vi "SetPropellerOutputPin.vi"(6 "error in (no error)":errorcluster, 8 "Pin Number":dbl, 9 "Value":bool, 10 "Dir":bool, 11 "SerialPortRef":T1) -> (0 "error out":errorcluster, 3 "SerialPortRef 2":T1)   [LabVIEW 2015]
uses:
  <vilib>/Rock Robotics/WPI/SerialPort/WPI_SerialPortRef.ctl
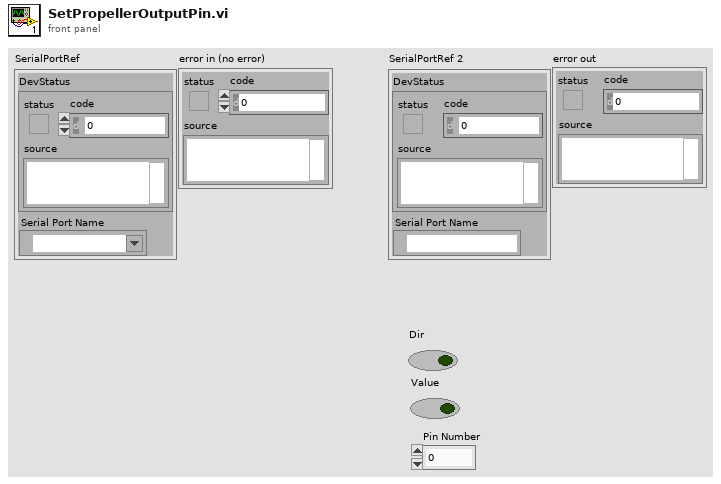
[diagram p1: front panel]
types:
  T1 = typedef "WPI_SerialPortRef.ctl" = cluster{"DevStatus":errorcluster, "Serial Port Name":refnum<visa-resource-name>}
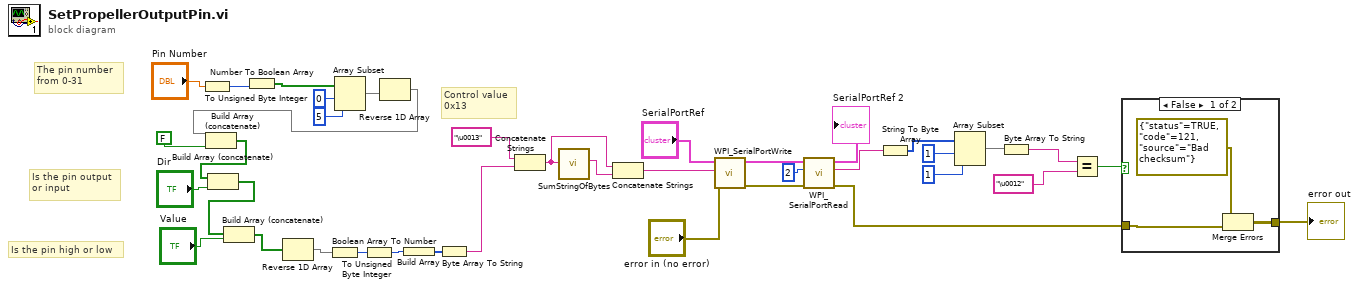
[diagram p0: block diagram]
diagram:
  # "The pin number\nfrom 0-31"
  # "Is the pin high or low"
  # "Is the pin output\nor input"
  # "Control value\n0x13"
  n1 = To Unsigned Byte Integer(number="Pin Number") -> (unsigned 8bit integer=w31:u8)
  n2 = Number To Boolean Array(number=w31) -> (Boolean array=w24:bool[])
  n3 = Array Subset(array=w24, index=0, length=5) -> (w25:bool[])
  n4 = Reverse 1D Array(array=w25) -> (reversed array=w23:bool[])
  n5 = Build Array (concatenate)(w23, FALSE ("new element/subarray")) -> (w21:bool[])
  n6 = Build Array (concatenate)(w21, "Dir") -> (w18:bool[])
  n7 = Build Array (concatenate)(w18, "Value") -> (w17:bool[])
  n8 = Reverse 1D Array(array=w17) -> (reversed array=w16:bool[])
  n9 = Boolean Array To Number(Boolean array=w16) -> (number=w30:u32)
  n10 = To Unsigned Byte Integer(number=w30) -> (unsigned 8bit integer=w29:u8)
  n11 = Build Array(w29) -> (w28:u8[])
  n12 = Byte Array To String(unsigned byte array=w28) -> (string=w14:string)
  n13 = Concatenate Strings("\u0013" ("Buffer"), w14) -> (w12:string)
  n14 = call "SumStringOfBytes.vi"("String Of Bytes"=w12) -> ("SumAsString"=w13:string)  [unwired: 10 in]
  n15 = Concatenate Strings(w12, w13) -> (w11:string)
  n16 = call <vilib>:"WPI_SerialPortWrite.vi"("error in (no error)"="error in (no error)", "Buffer"=w11, "SerialPortRef"="SerialPortRef") -> ("error out"=w35:errorcluster, "SerialPortRef"=w36:T1)  [unwired: 6 in, 1 out]
  n17 = call <vilib>:"WPI_SerialPortRead.vi"("error in (no error)"=w35, "Num Bytes to Read"=u32 2, "SerialPortRef"=w36) -> ("error out"=w9:errorcluster, "Buffer"=w7:string, "SerialPortRef"=→"SerialPortRef 2":T1)  [unwired: 6 in]
  n18 = String To Byte Array(string=w7) -> (unsigned byte array=w10:u8[])
  n19 = Array Subset(array=w10, index=1, length=1) -> (w3:u8[])
  n20 = Byte Array To String(unsigned byte array=w3) -> (string=w2:string)
  n21 = Equal?(x=w2, y="\u0012" ("Buffer")) -> (x = y?=w6:bool)
  n22 = case shown="False" w6 {
    tunnel: w9 -> [w40 w42]
    tunnel: [w39 w42] -> w8
    frame False {
      n23 = Merge Errors(errorcluster {"status"=TRUE, "code"=121, "source"="Bad checksum"} ("error in"), w40) -> (w39:errorcluster)
    }
    frame True {
    }
  }
  "error out" <- w8
